vi "ClimbStateMachine.vi"(6 "PullLS":bool, 8 "ReachLS":bool, 9 "ClimbEncoder":dbl, 10 "Array":bool[](array[boolean]), 11 "Cancel":bool) -> (1 "MotorOutput":dbl, 2 "ClimbStates":T1)   [LabVIEW 2023]
uses:
  ClimbStates.ctl
panel:
  # "ClimbRest"
  # "ClimbReach"
  # "ClimbPull"
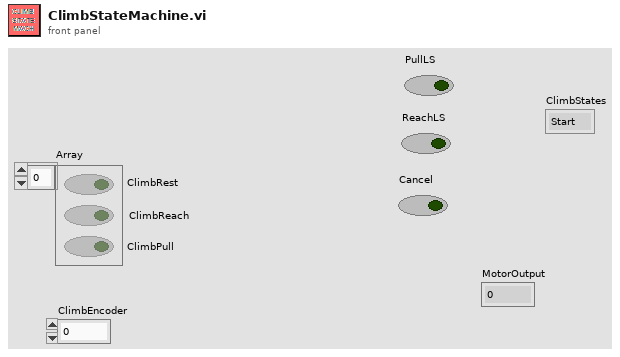
[diagram p1: front panel]
types:
  T1 = typedef "ClimbStates.ctl" = enum16{"Start", "WaitForCommands", "ClimbRest", "ClimbReach", "ClimbPull"}
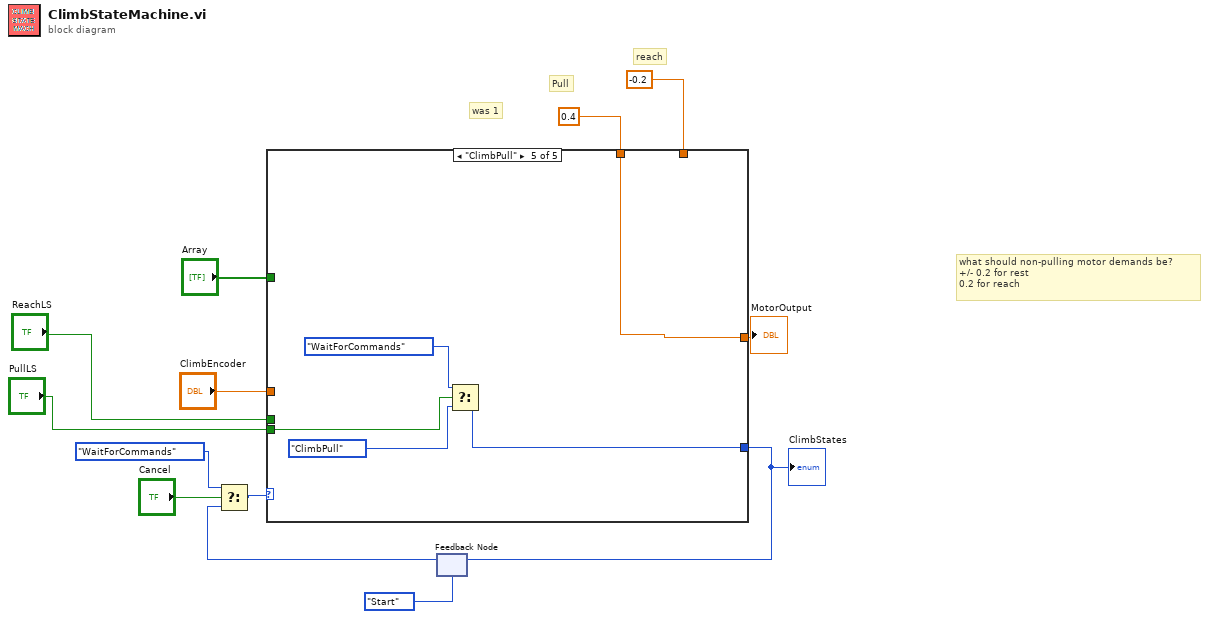
[diagram p0: block diagram]
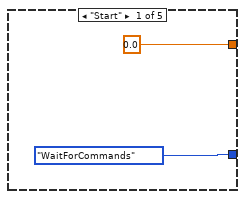
[diagram p2: hidden frame]
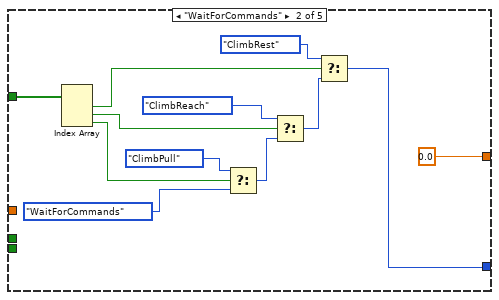
[diagram p3: hidden frame]
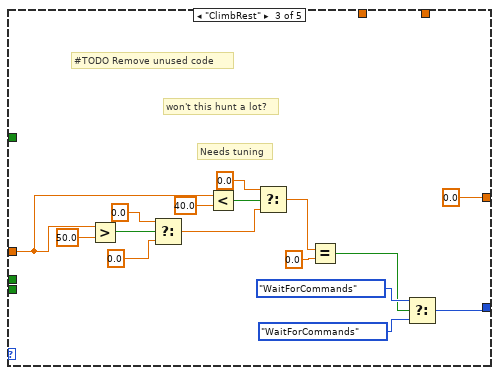
[diagram p4: hidden frame]
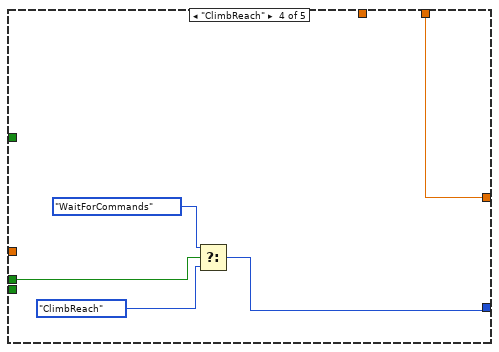
[diagram p5: hidden frame]
diagram:
  # "was 1"
  # "reach"
  # "Pull"
  # "what should non-pulling motor demands be?\n+/- 0.2 for rest\n0.2 for reach"
  n1 = feedback #1(ClimbStates."Start") -> (w8:T1)
  n2 = Select(t=ClimbStates."WaitForCommands", s="Cancel", f=w8) -> (s? t:f=w6:T1)
  n3 = case shown="\"ClimbPull\"" w6 {
    tunnel: [0.0 0.0 0.0 w44 w49] -> w12
    tunnel: "Array" -> [_ w26 _ _ _]
    tunnel: "ClimbEncoder" -> [_ _ w33 _ _]
    tunnel: [ClimbStates."WaitForCommands" w16 w38 w46 w52] -> w3
    tunnel: "ReachLS" -> [_ _ _ w45 _]
    tunnel: "PullLS" -> [_ _ _ _ w50]
    tunnel: 0.4 -> [_ _ _ _ w49]
    tunnel: -0.2 -> [_ _ _ w44 _]
    frame "Start" {
    }
    frame "WaitForCommands" {
      n4 = Index Array(array=w26) -> (element #1=w25:bool, element #2=w24:bool, element #3=w21:bool)  [unwired: 3 in]
      n5 = Select(t=ClimbStates."ClimbPull", s=w21, f=ClimbStates."WaitForCommands") -> (s? t:f=w22:T1)
      n6 = Select(t=ClimbStates."ClimbReach", s=w24, f=w22) -> (s? t:f=w23:T1)
      n7 = Select(t=ClimbStates."ClimbRest", s=w25, f=w23) -> (s? t:f=w16:T1)
    }
    frame "ClimbRest" {
      # "#TODO Remove unused code"
      # "Needs tuning"
      # "won't this hunt a lot?"
      n8 = Greater?(x=w33, y=50.0) -> (0:w43:bool)
      n9 = Select(t=0.0, s=w43, f=0.0) -> (s? t:f=w35:dbl)
      n10 = Less?(x=w33, y=40.0) -> (x < y?=w34:bool)
      n11 = Select(t=0.0, s=w34, f=w35) -> (s? t:f=w30:dbl)
      n12 = Equal?(x=w30, y=0.0) -> (x = y?=w29:bool)
      n13 = Select(t=ClimbStates."WaitForCommands", s=w29, f=ClimbStates."WaitForCommands") -> (s? t:f=w38:T1)
    }
    frame "ClimbReach" {
      n14 = Select(t=ClimbStates."WaitForCommands", s=w45, f=ClimbStates."ClimbReach") -> (s? t:f=w46:T1)
    }
    frame "ClimbPull" {
      n15 = Select(t=ClimbStates."WaitForCommands", s=w50, f=ClimbStates."ClimbPull") -> (s? t:f=w52:T1)
    }
  }
  "MotorOutput" <- w12
  "ClimbStates" <- w3
  n16 = feedback-in #1(w3) -> ()
